vi "INI.GetSettings.vi"(8 "error in (no error)":errorcluster) -> (0 "error out":errorcluster, 3 "INI.Settings":T1={"Build Location"=path "C:/Simple Sequence Editor/SequenceRepo", "LoggingLocation"=path ""})   [LabVIEW 2013, in "Simple Sequence Editor.lvlib"]
uses:
  Simple Sequence Editor.lvlib
  Types/INI.Settings
  Constants.vi
  <vilib>/Utility/config.llb/Read Key (Path).vi
  <vilib>/Utility/config.llb/Write Key (Path).vi
  <vilib>/Utility/config.llb/NI_LVConfig.lvlib
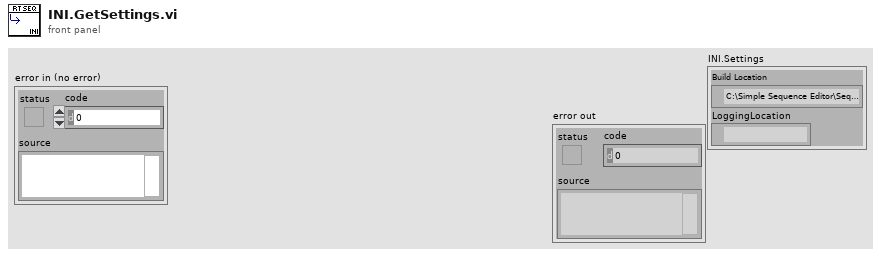
[diagram p1: front panel]
types:
  T1 = typedef "Simple Sequence Editor.lvlib/INI.Settings" = cluster{"Build Location":path, "LoggingLocation":path}
  T2 = typedef "NI_LVConfig.lvlib/Config Data RefNum.ctl" = refnum<k1>
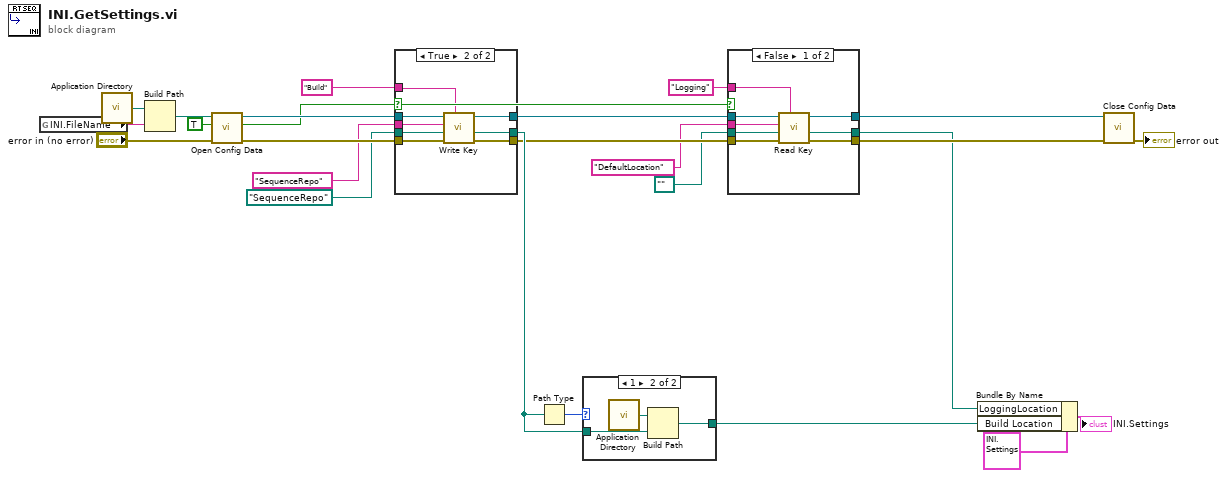
[diagram p0: block diagram]
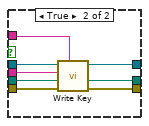
[diagram p2: hidden frame]
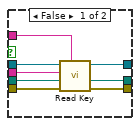
[diagram p3: hidden frame]
diagram:
  n1 = global read "Constants.vi" "INI.FileName"() -> (w16:string)
  n2 = call <vilib>:"Application Directory.vi"() -> ("Application Directory"=w18:path)
  n3 = Build Path(base path=w18, name or relative path=w16) -> (appended path=w17:path)
  n4 = call <vilib>:"Open Config Data.vi"("error in (no error)"="error in (no error)", "create file if necessary (T)"=TRUE, "configuration file path"=w17) -> ("error out"=w24:errorcluster, "file created?"=w7:bool, "refnum"=w25:T2)  [unwired: 6 in]
  n5 = case shown="True" w7 {
    tunnel: w25 -> [w33 w38]
    tunnel: w24 -> [w32 w40]
    tunnel: [w31 w36] -> w9
    tunnel: [w30 w34] -> w4
    tunnel: "Build" ("section") -> [w29 w37]
    tunnel: "SequenceRepo" ("key") -> [w28 w39]
    tunnel: path "SequenceRepo" ("default value") -> [w27 w35]
    tunnel: [w26 w35] -> w19
    frame False {
      n6 = call-poly <vilib>:"Read Key.vi"("section"=w29, "error in (no error)"=w32, "default value"=w27, "key"=w28, "refnum"=w33) -> ("error out"=w31:errorcluster, "value"=w26:path, "refnum out"=w30:T2)  [unwired: 3 in, 1 out]
    }
    frame True {
      n7 = call-poly <vilib>:"Write Key.vi"("section"=w37, "error in (no error)"=w40, "value"=w35, "key"=w39, "refnum"=w38) -> ("error out"=w36:errorcluster, "refnum out"=w34:T2)  [unwired: 4 in, 1 out]
    }
  }
  n8 = Path Type(1:w19) -> (0:w20:i16)
  n9 = case shown="1" w20 {
    tunnel: w19 -> [w41 w43]
    tunnel: [w41 w42] -> w11
    frame 0, Default {
    }
    frame 1 {
      n10 = call <vilib>:"Application Directory.vi"() -> ("Application Directory"=w44:path)
      n11 = Build Path(base path=w44, name or relative path=w43) -> (appended path=w42:path)
    }
  }
  n12 = case shown="False" w7 {
    tunnel: w4 -> [w52 w57]
    tunnel: w9 -> [w51 w59]
    tunnel: [w50 w55] -> w8
    tunnel: [w49 w53] -> w3
    tunnel: "Logging" ("section") -> [w48 w56]
    tunnel: "DefaultLocation" ("key") -> [w47 w58]
    tunnel: path "" ("default value") -> [w46 w54]
    tunnel: [w45 w54] -> w1
    frame False {
      n13 = call-poly <vilib>:"Read Key.vi"("section"=w48, "error in (no error)"=w51, "default value"=w46, "key"=w47, "refnum"=w52) -> ("error out"=w50:errorcluster, "value"=w45:path, "refnum out"=w49:T2)  [unwired: 3 in, 1 out]
    }
    frame True {
      n14 = call-poly <vilib>:"Write Key.vi"("section"=w56, "error in (no error)"=w59, "value"=w54, "key"=w58, "refnum"=w57) -> ("error out"=w55:errorcluster, "refnum out"=w53:T2)  [unwired: 4 in, 1 out]
    }
  }
  n15 = Bundle By Name(cluster=T1 {"Build Location"=path "C:/Simple Sequence Editor/SequenceRepo", "LoggingLocation"=path ""}, "LoggingLocation"=w1, "Build Location"=w11) -> (→"INI.Settings":T1)
  n16 = call <vilib>:"Close Config Data.vi"("error in (no error)"=w8, "refnum"=w3) -> ("error out"=→"error out":errorcluster)  [unwired: 8 in, 1 out]
